vi "ConnectTo.vi"(8 "error in":errorcluster, 11 "AdapterIn":T1) -> (0 "error out":errorcluster, 3 "CanHandleOut":T2)   [LabVIEW 2011, in "Konvolucio MCAN120803.lvlib"]
doc: "Connecting to a specific adapter."
uses:
  <instrlib>/Konvolucio MCAN120803/Konvolucio MCAN120803.lvlib
  <instrlib>/Konvolucio MCAN120803/Types/CanHandleType.ctl
  C:/Program Files/National Instruments/LabVIEW 2011/instr.lib/Konvolucio MCAN120803/Private/Konvolucio.MCAN120803.API.dll
  Private/Konvolucio.MCAN120803.API.dll
  <instrlib>/Konvolucio MCAN120803/Types/AdapterItemType.ctl
  <instrlib>/Konvolucio MCAN120803/Types/StateType.ctl
  <instrlib>/Konvolucio MCAN120803/Public/Attributes/AttrGetState.vi
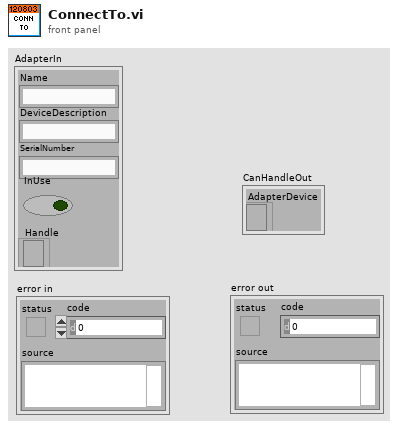
[diagram p1: front panel]
types:
  T1 = typedef "Konvolucio MCAN120803.lvlib/AdapterItemType.ctl" = cluster{"Name":string, "DeviceDescription":string, "SerialNumber":string, "InUse":bool, "Handle":refnum<k24>}
  T2 = typedef "Konvolucio MCAN120803.lvlib/CanHandleType.ctl" = cluster{"AdapterDevice":refnum<k24>}
  T3 = typedef "Konvolucio MCAN120803.lvlib/StateType.ctl" = enum16{"SDEV_NONE", "SDEV_START", "SDEV_STOP", "SDEV_RESET", "SDEV_FAIL", "SDEV_IDLE"}
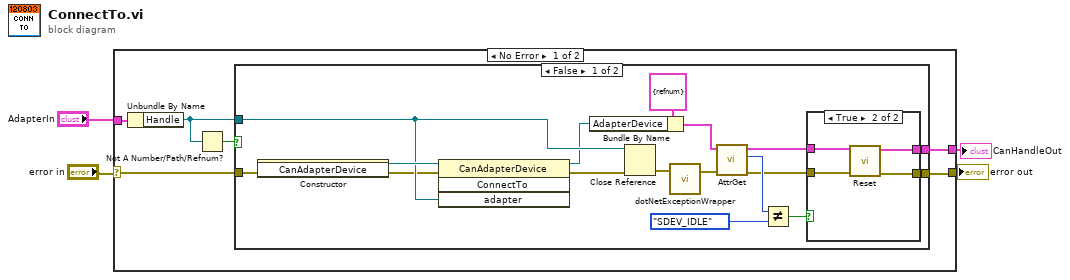
[diagram p0: block diagram]
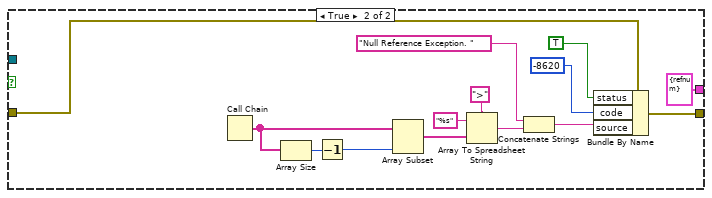
[diagram p3: hidden frame]
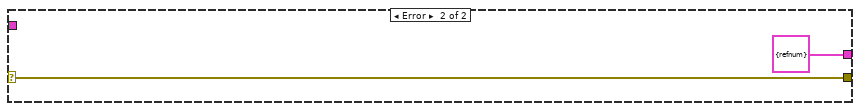
[diagram p4: hidden frame]
diagram:
  n1 = case shown="No Error" "error in" {
    selector: "error in" -> [w7 w49]
    tunnel: "AdapterIn" -> [w10 _]
    tunnel: [w8 w49] -> w3
    tunnel: [w9 T2 {"AdapterDevice"=refnum} ("MCanHandleOut")] -> w2
    frame No Error {
      n2 = Unbundle By Name(w10) -> ("Handle"=w6:refnum<k24>)
      n3 = Not A Number/Path/Refnum?(number/path/refnum=w6) -> (NaN/Path/Refnum?=w5:bool)
      n4 = case shown="False" w5 {
        tunnel: w6 -> [w14 _]
        tunnel: [w19 T2 {"AdapterDevice"=refnum} ("MCanHandleOut")] -> w9
        tunnel: [w18 w36] -> w8
        tunnel: w7 -> [w15 w35]
        frame False {
          n5 = constructor class="CanAdapterDevice"(error in=w15) -> (reference out=w27:refnum<k24>, error out=w13:errorcluster)  [unwired: 2 in, 1 out]
          n6 = invoke class="CanAdapterDevice" method="ConnectTo"(reference=w27, error in=w13, "adapter"=w14) -> (reference out=w12:refnum<k24>, error out=w11:errorcluster)  [unwired: 1 in, 2 out]
          n7 = Bundle By Name(cluster=T2 {"AdapterDevice"=refnum}, "AdapterDevice"=w12) -> (w25:T2)
          n8 = Close Reference(reference=w14, error in (no error)=w11) -> (error out=w17:errorcluster)
          n9 = call <instrlib>:"dotNetExceptionWrapper.vi"("error in"=w17) -> ("error out"=w16:errorcluster)  [unwired: 2 in]
          n10 = call-poly <instrlib>:"AttrGet.vi"("error in"=w16, "CanHandleIn"=w25) -> ("error out"=w21:errorcluster, "State"=w23:T3, "CanHandleOut"=w20:T2)  [unwired: 7 in]
          n11 = Not Equal?(x=w23, y=StateType."SDEV_IDLE") -> (x != y?=w22:bool)
          n12 = case shown="True" w22 {
            tunnel: w21 -> [w28 w33]
            tunnel: w20 -> [w29 w32]
            tunnel: [w29 w31] -> w19
            tunnel: [w28 w30] -> w18
            frame False {
            }
            frame True {
              n13 = call <instrlib>:"Reset.vi"("error in"=w33, "CanHandleIn"=w32) -> ("error out"=w30:errorcluster, "CanHandleOut"=w31:T2)  [unwired: 8 in]
            }
          }
        }
        frame True {
          n14 = Call Chain() -> (call chain=w45:string[])
          n15 = Array Size(array=w45) -> (size(s)=w46:i32)
          n16 = Decrement(x=w46) -> (x-1=w47:i32)
          n17 = Array Subset(array=w45, length=w47) -> (w44:string[])  [unwired: 1 in]
          n18 = Array To Spreadsheet String(delimiter (Tab)=">", array=w44, 3:"%s" ("format string")) -> (spreadsheet string=w39:string)
          n19 = Concatenate Strings("Null Reference Exception. " ("source"), w39) -> (w37:string)
          n20 = Bundle By Name(cluster=w35, "status"=TRUE, "code"=-8620, "source"=w37) -> (w36:errorcluster)
        }
      }
    }
    frame Error {
    }
  }
  "error out" <- w3
  "CanHandleOut" <- w2
